vi "Msg.vi"(7 "LVCAM in":refnum<class "LVCAM.lvclass">, 11 "LVCAM Destroy Self Msg in":refnum<class "LVCAM Destroy Self Msg.lvclass">) -> (0 "error out":errorcluster, 1 "Destroyed Self?":bool, 5 "LVCAM out":refnum<class "LVCAM.lvclass">)   [LabVIEW 2021, in "LVCAM Destroy Self.lvlib" / "LVCAM Destroy Self Msg.lvclass"]
uses:
  LVCAM Destroy Self Msg.lvclass
  LVCAM/LVCAM/LVCAM.lvclass
  LVCAM Destroy Self/LVCAM Destroy Self.lvclass
  LVCAM Destroy Self Msg.lvclass/LVCAM Destroy Self Msg.ctl
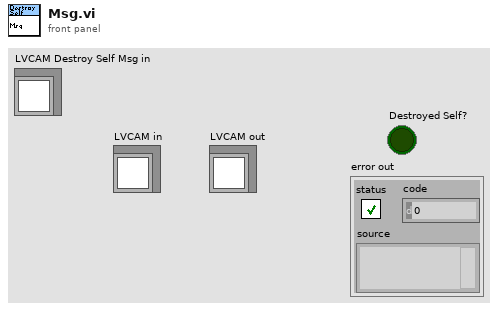
[diagram p1: front panel]
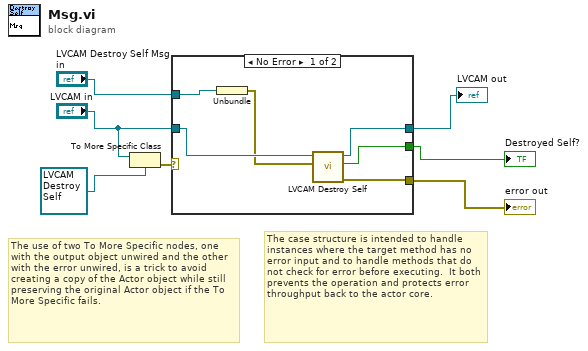
[diagram p0: block diagram]
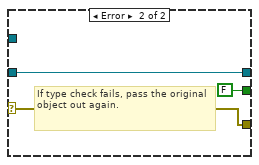
[diagram p2: hidden frame]
diagram:
  # "The use of two To More Specific nodes, one with the output object unwired and the other with the error unwired, is a trick to avoid creating a copy of the Actor object while still preserving the original Actor object if the To More Specific fails."
  # "The case structure is intended to handle instances where the target method has no error input and to handle methods that do not check for error before executing.  It both prevents the operation and protects error throughput back to the actor core."
  n1 = To More Specific Class(target class=refnum<class "LVCAM Destroy Self.lvclass"> refnum ("Destroy.lvlib:Destroy.lvclass"), reference="LVCAM in") -> (error out=w7:errorcluster)  [unwired: 1 in, 1 out]
  n2 = case shown="No Error" w7 {
    selector: w7 -> [_ w16]
    tunnel: [w9 w16] -> w6
    tunnel: [w8 w15] -> w4
    tunnel: "LVCAM in" -> [w13 w15]
    tunnel: "LVCAM Destroy Self Msg in" -> [w12 _]
    tunnel: [w10 FALSE ("Destroyed Self?")] -> w1
    frame No Error {
      n3 = Unbundle(w12) -> (w11:errorcluster)
      n4 = call-dynamic "LVCAM Destroy Self.vi"("Error"=w11, "LVCAM Destroy Self in"=w13) -> ("error out"=w9:errorcluster, "Destroyed Self?"=w10:bool, "LVCAM Destroy Self out"=w8:refnum<class "LVCAM.lvclass">)  [unwired: 7 in]
    }
    frame Error {
      # "If type check fails, pass the original object out again."
    }
  }
  "error out" <- w6
  "Destroyed Self?" <- w1
  "LVCAM out" <- w4
